vi "test so.vi"() -> ()   [LabVIEW 2025]
uses:
  <vilib>/Platform/TimedLoop/XDataNode/timing_clust.ctl
  <vilib>/Platform/TimedLoop/XDataNode/nitl_modes.ctl
  <vilib>/Platform/TimedLoop/XDataNode/wakeup.ctl
  <vilib>/platform/TimedLoop/XDataNode/XDataNode.xnode
  <vilib>/Platform/TimedLoop/XDataNode/XDNodeRunTimeDep.lvlib
  home/lvuser/natinst/waveform_gen.so
panel:
  in  "stop":bool
  in  "Generate":bool
  in  "samples":i32=4410
  out "Waveform Graph":dbl[](graph)
  in  "dt":dbl=2.26757e-05
  in  "Amplitude":dbl=1.0
  in  "Freq Stop":dbl=300.0
  in  "Freq Start":dbl=100.0
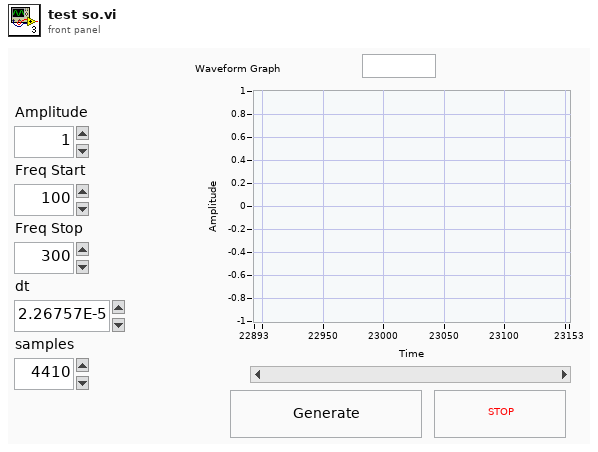
[diagram p1: front panel]
types:
  T1 = typedef "XDNodeRunTimeDep.lvlib/timing_clust.ctl" = cluster{"Expected End [f-1]":u64, "Actual End [f-1]":u64, "Finished Late? [f-1]":bool, "Expected End [i-1]":u64, "Actual End [i-1]":u64, "Finished Late? [i-1]":bool, "Expected Start [i]":u64, "Actual Start [i]":u64, "Expected Start [f]":u64, "Actual Start [f]":u64, "Source Name":string, "Structure Name":string, "Period":i64, "Deadline":i64, "Offset":i64, "Start":i64, "Priority":i32, "Timeout":i32, "Mode":T2, "Wakeup Reason":T3, "Error":errorcluster, "Source Type":string, "Secondary Source Type":string, "Global End Time":u64, "Global Start Time":u64, "Frame Duration":u64, "Iteration Duration":u64, "Assigned CPU":i32, "I/O Scan Engine Mode":u32}
  T2 = typedef "XDNodeRunTimeDep.lvlib/nitl_modes.ctl" = enum32{"No Change", "Process missed periods, maintain original phase", "Discard missed periods, maintain original phase", "Process missed periods, ignore original phase", "Discard missed periods, ignore original phase"}
  T3 = typedef "XDNodeRunTimeDep.lvlib/wakeup.ctl" = enum32{"Normal", "Aborted", "Asynchronous wakeup", "Timing source error", "Timed loop error", "Timeout"}
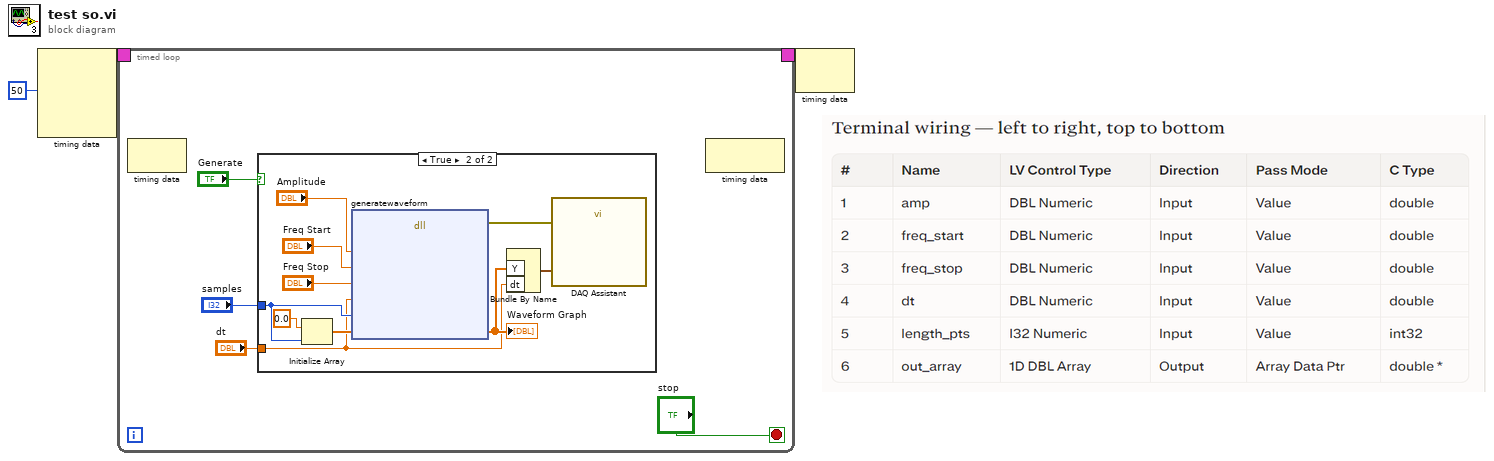
[diagram p0: block diagram]
diagram:
  n1 = node-c288(i64 50 ("Period")) -> (w3:T1)  [unwired: 3 in]
  n2 = timed-loop {
    timing: w3 -> [_]
    timing-out: [_] -> w2
    stop <- "stop" stop-if-true
    n3 = node-c288() -> ()  [unwired: 1 in, 1 out]
    n4 = case shown="True" "Generate" {
      tunnel: "samples" -> [_ w10]
      tunnel: "dt" -> [_ w9]
      frame False {
      }
      frame True {
        n5 = Initialize Array(0.0 ("element"), w10) -> (w14:dbl[])
        n6 = dll-call lib="home/lvuser/natinst/waveform_gen.so" fn="generatewaveform"("amp"="Amplitude", "freq_start"="Freq Start", "freq_stop"="Freq Stop", "dt"=w9, "Length_pts"=w10, "out_array"=w14) -> (error out=w13:errorcluster, "out_array"=w12:dbl[])  [unwired: 9 in, 1 out]
        "Waveform Graph" <- w12
        n7 = Bundle By Name("Y"=w12, "dt"=w9) -> (w11:waveform(dbl))  [unwired: 1 in]
        n8 = call "DAQ Assistant"("data"=w11, "error in"=w13) -> ()  [unwired: 16 in, 2 out]
      }
    }
    n9 = node-c288() -> ()  [unwired: 1 in, 1 out]
  }
  n10 = node-c288(w2) -> ()  [unwired: 1 out]
